vi "Write Execution Time.vi"(8 "error in":errorcluster, 10 "Values in":dbl[](array[numeric]), 11 "Execution Unit in":refnum<class "Execution Unit.lvclass">) -> (0 "error out":errorcluster, 2 "Values out":dbl[](array[numeric]), 3 "Execution Unit out":refnum<class "Execution Unit.lvclass">)   [LabVIEW 2020, in "Ballard ARINC 429 Engine.lvlib" / "Implementation.lvlib" / "Execution Unit.lvclass"]
uses:
  Execution Unit.lvclass
  Execution Unit.lvclass/Execution Unit.ctl
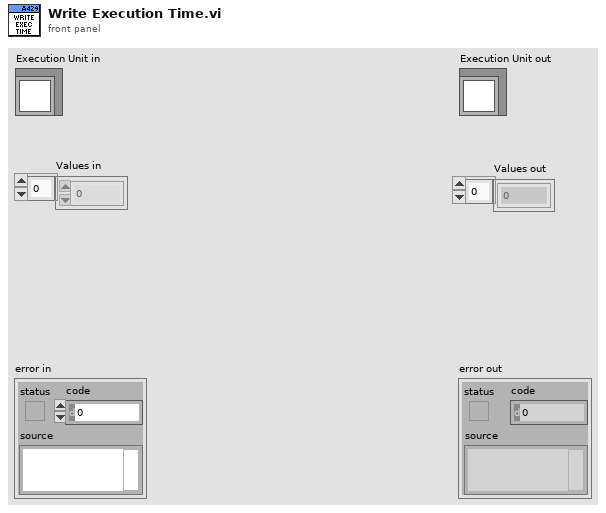
[diagram p1: front panel]
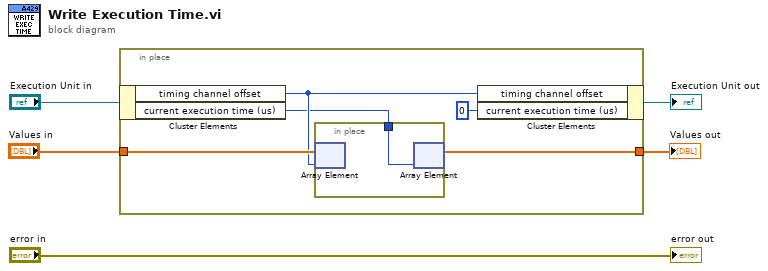
[diagram p0: block diagram]
diagram:
  n1 = in-place {
    in-place-border: "Values in" -> [w10]
    in-place-border: [w6] -> w2
    n2 = in-place-cluster #1("Execution Unit in") -> ("timing channel offset"=w9:i64, "current execution time (us)"=w8:u32)
    n3 = in-place {
      in-place-border: w8 -> [w11]
      n4 = in-place-array #2(w10, w9) -> ()  [unwired: 1 out]
      n5 = in-place-array #2(w11) -> (w6:dbl[])  [unwired: 1 out]
    }
    n6 = in-place-cluster #1("timing channel offset"=w9, "current execution time (us)"=u32 0) -> (→"Execution Unit out":refnum<class "Execution Unit.lvclass">)
  }
  "Values out" <- w2
  "error out" <- "error in"
